vi "Write Outgoing Bytes.vi"(8 "error in (no error)":errorcluster, 9 "timeout ms (2000)":i32=2000, 10 "Bytes":u8[](array[numeric]) format="%08b", 11 "Connection.TCP-TLS in":refnum<class "Connection.TCP-TLS.lvclass">) -> (0 "error out":errorcluster, 3 "Connection.TCP-TLS out":refnum<class "Connection.TCP-TLS.lvclass">)   [LabVIEW 2020]
uses:
  Connection.TCP-TLS.lvclass
  Connection.TCP-TLS.lvclass/Connection.TCP-TLS.ctl
  C:/Program Files (x86)/National Instruments/LabVIEW 2020/vi.lib/LabVIEW Open Source Project/MQTT TCP Connection/MQTT_TCP/Connection/TCPConnection.lvclass
  C:/Program Files (x86)/National Instruments/LabVIEW 2020/vi.lib/LabVIEW Open Source Project/MQTT Connection/MQTT_Connection/Connection/Connection.lvclass
  C:/Projects/LVOS/MQTT-Connection-TCP.TLS/source/Connection.SecuredTCP/Connection.TCP-TLS.lvclass
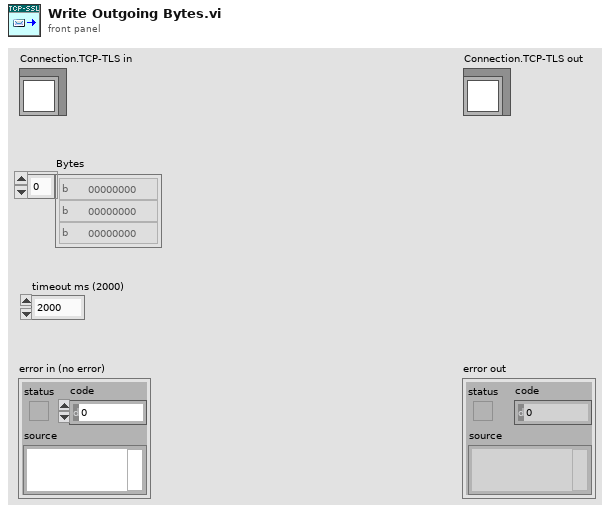
[diagram p1: front panel]
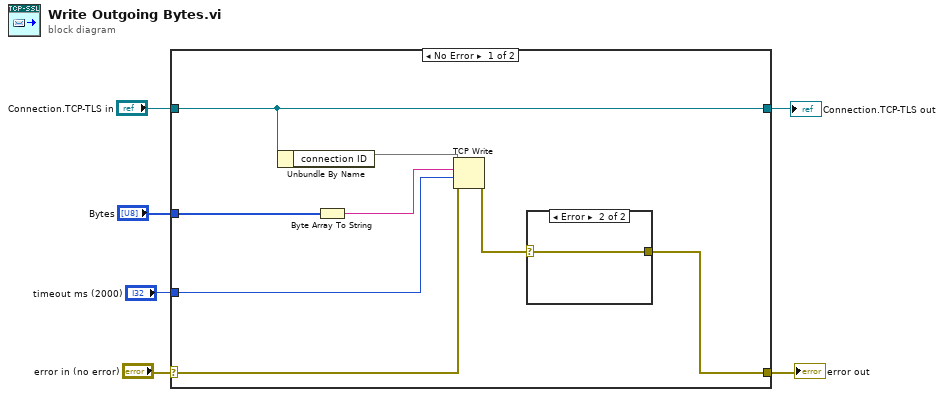
[diagram p0: block diagram]
diagram:
  n1 = case shown="No Error" "error in (no error)" {
    selector: "error in (no error)" -> [w10 w18]
    tunnel: [w8 w18] -> w1
    tunnel: [w14 w17] -> w2
    tunnel: "Connection.TCP-TLS in" -> [w14 w17]
    tunnel: "Bytes" -> [w12 _]
    tunnel: "timeout ms (2000)" -> [w7 _]
    frame No Error {
      n2 = Unbundle By Name(w14) -> ("connection ID"=w13)
      n3 = Byte Array To String(unsigned byte array=w12) -> (string=w11:string)
      n4 = TCP Write(connection ID=w13, data in=w11, error in (no error)=w10, 9:w7) -> (error out=w9:errorcluster)  [unwired: 2 out]
      n5 = case shown="Error" w9 {
        selector: w9 -> [w15 w16]
        tunnel: [w15 w16] -> w8
        frame No Error {
        }
        frame Error {
        }
      }
    }
    frame Error {
    }
  }
  "error out" <- w1
  "Connection.TCP-TLS out" <- w2
